vi "Boolean String to Boolean.vi"(8 "error in (no error)":errorcluster, 11 "String":string) -> (0 "error out":errorcluster, 3 "Boolean":bool)   [LabVIEW 2013]
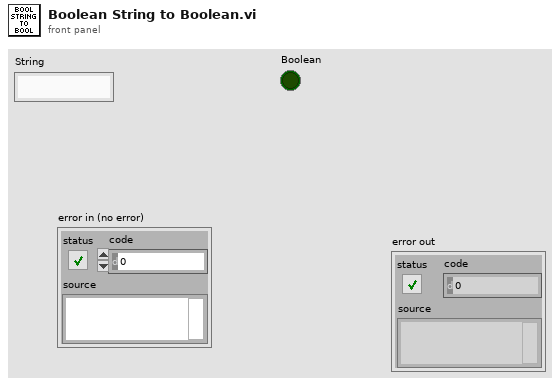
[diagram p1: front panel]
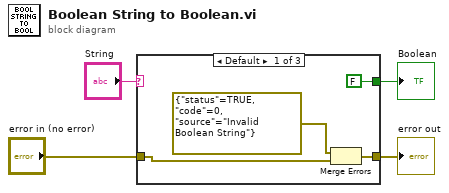
[diagram p0: block diagram]
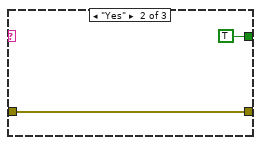
[diagram p2: hidden frame]
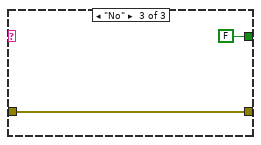
[diagram p3: hidden frame]
diagram:
  n1 = case shown="Default" "String" {
    tunnel: [FALSE TRUE FALSE] -> w3
    tunnel: "error in (no error)" -> [w7 w9 w11]
    tunnel: [w6 w9 w11] -> w1
    frame Default {
      n2 = Merge Errors(errorcluster {"status"=TRUE, "code"=0, "source"="Invalid Boolean String"} ("error in"), w7) -> (w6:errorcluster)
    }
    frame "Yes" {
    }
    frame "No" {
    }
  }
  "Boolean" <- w3
  "error out" <- w1
